vi "Get Pane Origin.vi"(8 "error in":errorcluster, 11 "VI Ref":refnum<vi>) -> (0 "error out":errorcluster, 2 "Pane Origin":T1[](array[typedef]), 3 "VI Ref":refnum<vi>)   [LabVIEW 2014]
doc: "Get the origin of all panes in the FP."
uses:
  <vilib>/Utility/miscctls.llb/LVPointTypeDef.ctl
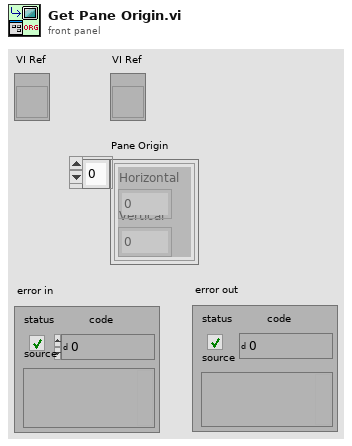
[diagram p1: front panel]
types:
  T1 = typedef "LVPointTypeDef.ctl" = cluster{"Horizontal":i16, "Vertical":i16}
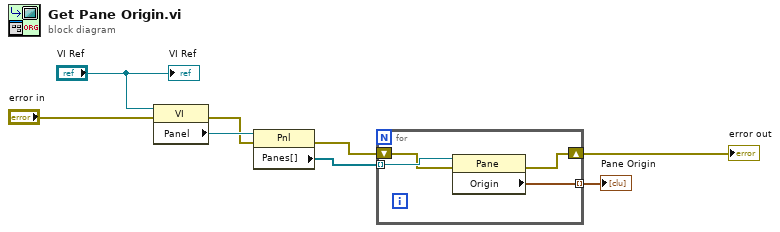
[diagram p0: block diagram]
diagram:
  n1 = property class="VI"(reference="VI Ref", error in="error in") -> (error out=w4:errorcluster, "Panel"=w7:refnum<vi>)  [unwired: 1 out]
  n2 = property class="Pnl"(reference=w7, error in=w4) -> (error out=w5:errorcluster, "Panes[]"=w6:refnum<vi>[])  [unwired: 1 out]
  n3 = for {
    tunnel: w6 -> [w12] mode=indexing
    tunnel: [w11] -> w3 mode=indexing
    shift-right: [w9] -> w2
    shift-left: w5 -> [w10]
    n4 = property class="Pane"(reference=w12, error in=w10) -> (error out=w9:errorcluster, "Origin"=w11:T1)  [unwired: 1 out]
  }
  "Pane Origin" <- w3
  "error out" <- w2
  "VI Ref" <- "VI Ref"
